vi "LINX Tasks.vi"() -> ()   [LabVIEW 2020]
doc: "This VI reads analog data from the DMA FIFO and converts it into readable signals and timestamps."
uses:
  Type Definitions/Payload Class.ctl
  Type Definitions/Enum - Data.ctl
  <vilib>/platform/TimedLoop/XDataNode/XDataNode.xnode
  <vilib>/Platform/TimedLoop/XDataNode/timing_clust.ctl
  <vilib>/Platform/TimedLoop/XDataNode/XDNodeRunTimeDep.lvlib
  <vilib>/Platform/TimedLoop/XDataNode/wakeup.ctl
  <vilib>/Platform/TimedLoop/XDataNode/nitl_modes.ctl
  <vilib>/MediaMongrels/LINX Raspberry Pi Addons/ADS1256 ADC/Channel Selection.ctl
  <vilib>/MediaMongrels/LINX Raspberry Pi Addons/LINX-DAC8552/Channel Select.ctl
  <vilib>/MediaMongrels/LINX Raspberry Pi Addons/LINX-DAC8552/Power Down Mode.ctl
  Type Definitions/Analog Output Command.ctl
  Type Definitions/Digital Output Command.ctl
  Type Definitions/Digital Output Data.ctl
  Type Definitions/Analog Output Data.ctl
  <vilib>/MakerHub/LINX/Public/Peripherals/Digital/Digital Write 1 Chan.vi
  <vilib>/MakerHub/LINX/Public/Peripherals/Digital/Digital Read N Chans.vi
panel:
  out "output cluster":T1 {"Port 0" format="%08b"}
  out "Error Out 3":errorcluster
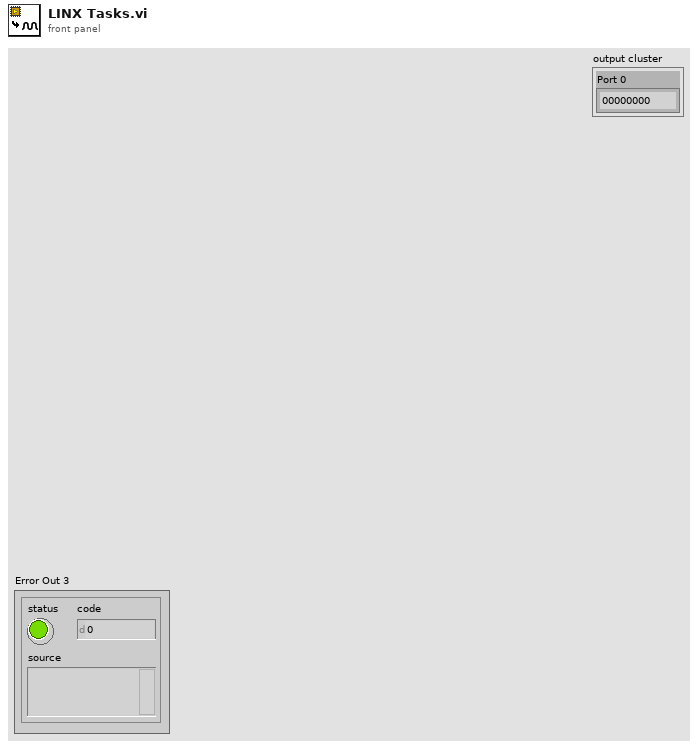
[diagram p1: front panel]
types:
  T1 = typedef "Digital Output Data.ctl" = cluster{"Port 0":u8}
  T2 = typedef "LINX-DAC8552.lvclass/Power Down Mode.ctl" = enum8{"On - Normal Operation", "Off - 1kOhm", "Off - 100kOhm", "Off - High Impedence"}
  T3 = typedef "LINX-DAC8552.lvclass/Channel Select.ctl" = enum8{"DAC A", "DAC B", "Both"}
  T4 = typedef "LINX Resources.ctl" = cluster{"LINX Resource":T5, "LINX SPI Data":refnum<class "LINX SPI.lvclass">, "ADS1256 Data":refnum<class "LINX-ADS1256.lvclass">, "DAC8552 Data":refnum<class "LINX-DAC8552.lvclass">}
  T5 = typedef "LMH-LINX.lvlib/LINX Ref.ctl" = cluster{"IO":T6, "Interface":T7, "LINX Device Config":T8}
  T6 = typedef "LMH-LINX.lvlib/Platform.ctl" = enum16{"Remote", "Local"}
  T7 = typedef "LMH-LINX.lvlib/Interface.ctl" = enum16{"Serial", "TCP"}
  T8 = typedef "LMH-LINX.lvlib/Device.lvlib/LINX Device Config.ctl" = cluster{"Interface":T7, "COM Port":refnum<visa-resource-name>, "TCP Configuration":T9, "Device Family":u8, "Device ID":u8, "Device Name":string, "TCP Ref":refnum<k5>, "Channels":T10}
  T9 = typedef "LMH-LINX.lvlib/Device.lvlib/TCP Config.ctl" = cluster{"IP Address":string, "Port":u16}
  T10 = typedef "LMH-LINX.lvlib/Channels.ctl" = cluster{"DI":u8[], "DO":u8[], "AI":u8[], "AO":u8[], "PWM":u8[], "QE":u8[], "UART":u8[], "I2C 2":u8[], "SPI":u8[], "CAN":u8[], "Servo":u8[], "AI Ref (V)":dbl, "AI Resolution (Bits)":u8, "AO Ref (V)":dbl, "AO Resolution (Bits)":u8}
  T11 = typedef "XDNodeRunTimeDep.lvlib/timing_clust.ctl" = cluster{"Expected End [f-1]":u64, "Actual End [f-1]":u64, "Finished Late? [f-1]":bool, "Expected End [i-1]":u64, "Actual End [i-1]":u64, "Finished Late? [i-1]":bool, "Expected Start [i]":u64, "Actual Start [i]":u64, "Expected Start [f]":u64, "Actual Start [f]":u64, "Source Name":string, "Structure Name":string, "Period":i64, "Deadline":i64, "Offset":i64, "Start":i64, "Priority":i32, "Timeout":i32, "Mode":T12, "Wakeup Reason":T13, "Error":errorcluster, "Source Type":string, "Secondary Source Type":string, "Global End Time":u64, "Global Start Time":u64, "Frame Duration":u64, "Iteration Duration":u64, "Assigned CPU":i32, "I/O Scan Engine Mode":u32}
  T12 = typedef "XDNodeRunTimeDep.lvlib/nitl_modes.ctl" = enum32{"No Change", "Process missed periods, maintain original phase", "Discard missed periods, maintain original phase", "Process missed periods, ignore original phase", "Discard missed periods, ignore original phase"}
  T13 = typedef "XDNodeRunTimeDep.lvlib/wakeup.ctl" = enum32{"Normal", "Aborted", "Asynchronous wakeup", "Timing source error", "Timed loop error", "Timeout"}
  T14 = typedef "Enum - Data.ctl" = enum16{"Analog Input Data", "Notification Data", "Analog Output Data", "Digital Output Data", "Command Ack", "Digital Input Data"}
  T15 = typedef "Payload Class.ctl" = enum16{"System State", "Parameters", "Metadata", "Software Monitor", "Data", "Commands"}
  T16 = typedef "Digital Output Command.ctl" = cluster{"DO Channel":u8, "State":bool}
  T17 = typedef "LINX-ADS1256.lvclass/Channel Selection.ctl" = enum16{"Differential 0-1", "Differential 2-3", "Differential 4-5", "Differential 6-7", "Single Ended 0", "Single Ended 1", "Single Ended 2", "Single Ended 3", "Single Ended 4", "Single Ended 5", "Single Ended 6", "Single Ended 7"}
  T18 = typedef "Analog Output Data.ctl" = cluster{"Bank 0":dbl[]}
  T19 = typedef "Analog Output Command.ctl" = cluster{"AO Channel":u8, "State":dbl}
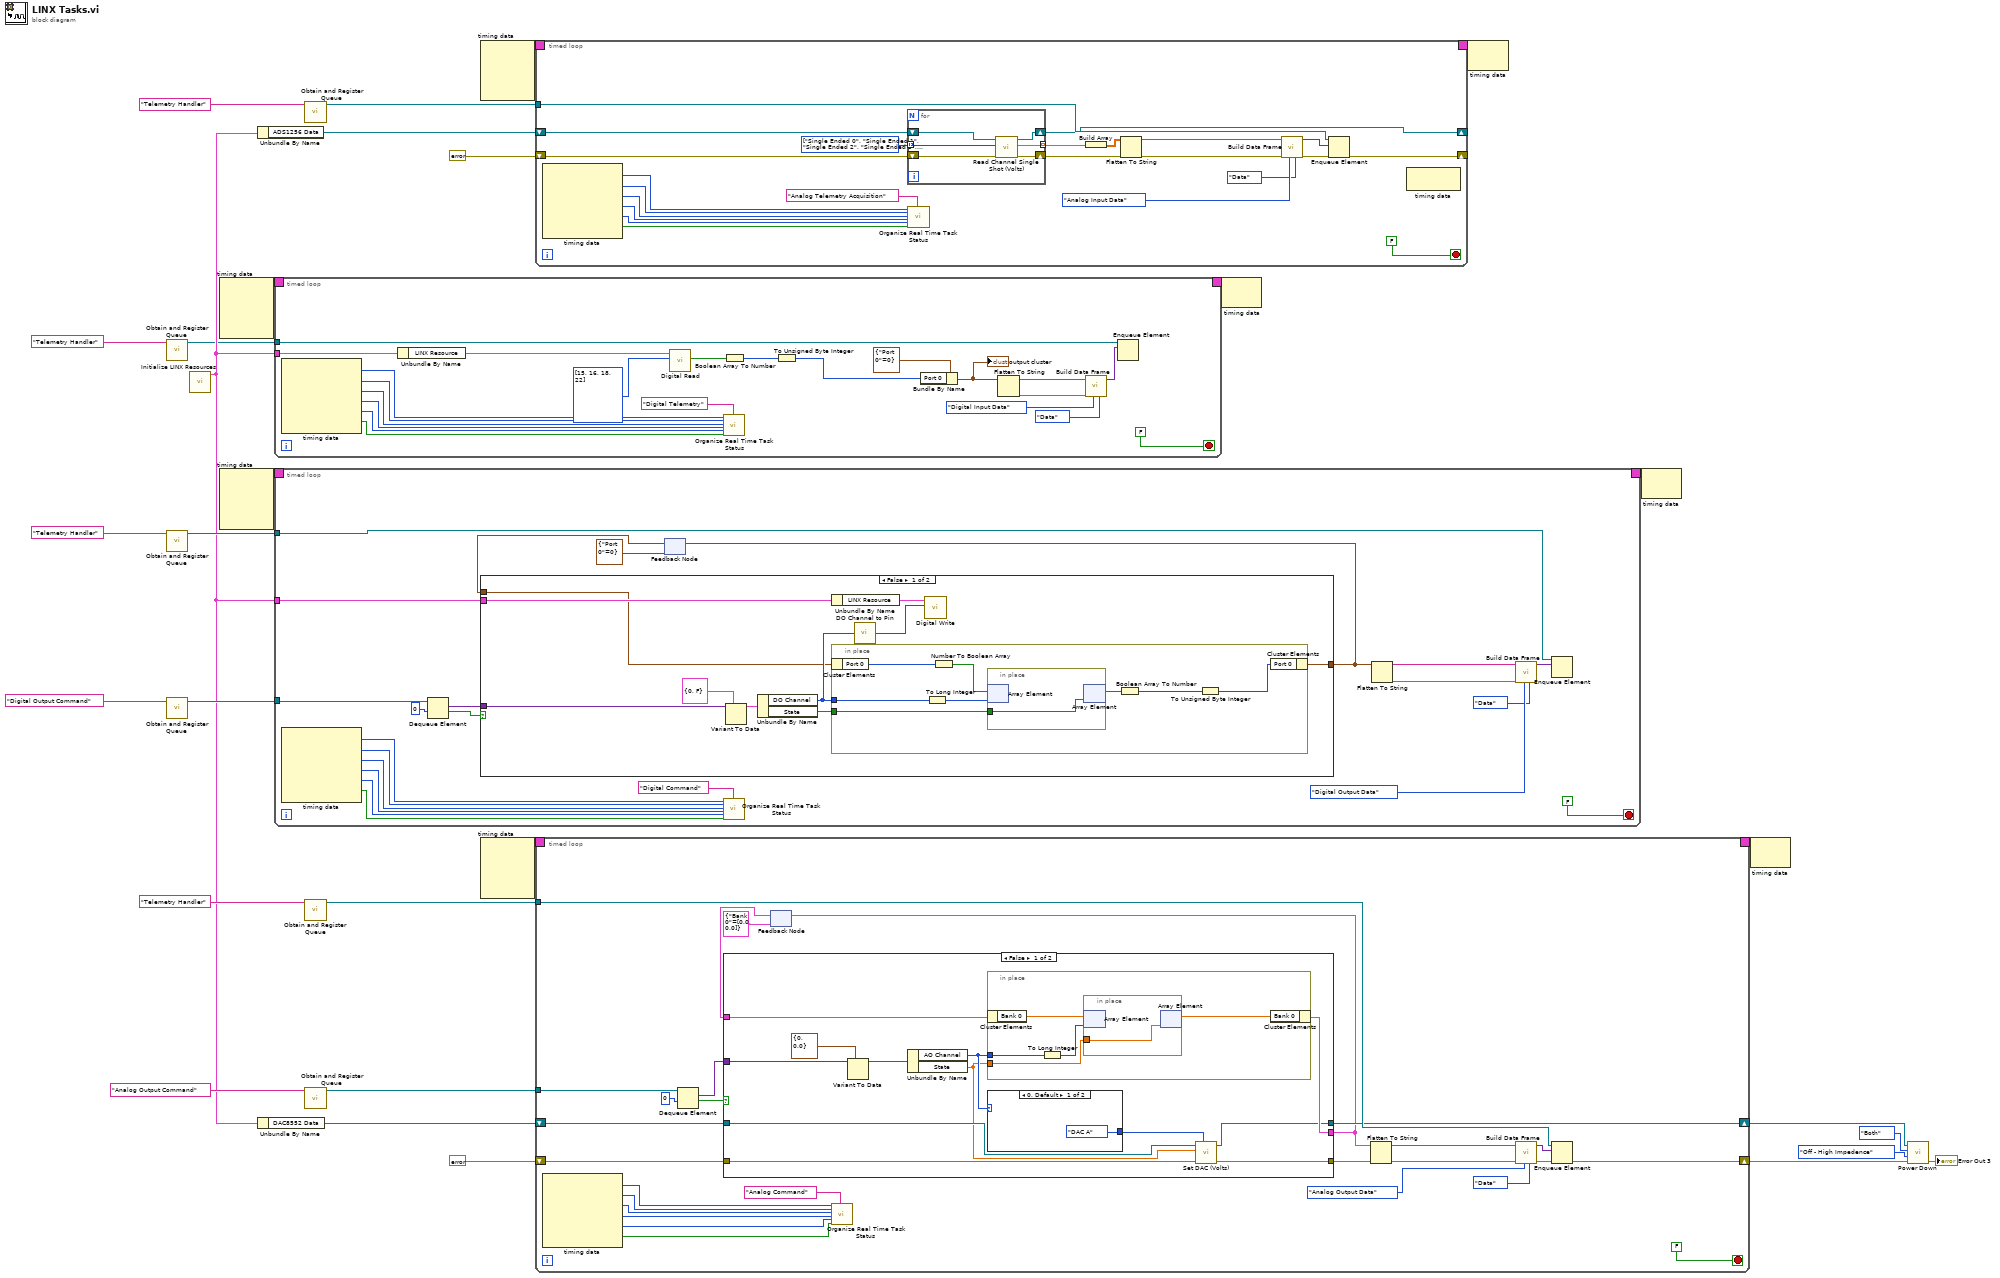
[diagram p0: block diagram]
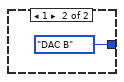
[diagram p2: hidden frame]
diagram:
  n1 = call "Obtain and Register Queue.vi"("name (unnamed)"="Telemetry Handler") -> ("Queue Out"=w1:refnum<queue>)  [unwired: 7 in, 3 out]
  n2 = call "Obtain and Register Queue.vi"("name (unnamed)"="Telemetry Handler") -> ("Queue Out"=w18:refnum<queue>)  [unwired: 7 in, 3 out]
  n3 = call "Obtain and Register Queue.vi"("name (unnamed)"="Digital Output Command") -> ("Queue Out"=w16:refnum<queue>)  [unwired: 7 in, 3 out]
  n4 = call "Initialize LINX Resources.vi"() -> ("LINX Resources"=w3:T4)  [unwired: 11 in]
  n5 = node-c288() -> (w5:T11)  [unwired: 4 in]
  n6 = node-c288() -> (w20:T11)  [unwired: 4 in]
  n7 = Unbundle By Name(w3) -> ("DAC8552 Data"=w24:refnum<class "LINX-DAC8552.lvclass">)
  n8 = Unbundle By Name(w3) -> ("ADS1256 Data"=w23:refnum<class "LINX-ADS1256.lvclass">)
  n9 = timed-loop {
    timing: w5 -> [_]
    timing-out: [_] -> w4
    tunnel: w1 -> [w38]
    tunnel: w3 -> [w44]
    stop <- FALSE stop-if-true
    n10 = node-c288() -> (w50:i32, w49:i32, w48:i64, w47:i64, w46:i64, w45:bool)  [unwired: 1 in]
    n11 = Unbundle By Name(w44) -> ("LINX Resource"=w37:T5)
    n12 = call-poly <vilib>:"Digital Read.vi"("DI Channels"=u8[] [15, 16, 18, 22] ("Array 3"), "LINX Resource"=w37) -> ("Values"=w35:bool[])  [unwired: 7 in, 2 out]
    n13 = call "Organize Real Time Task Status.vi"("Priority"=w50, "Processor"=w49, "Offset"=w48, "Iteration Duration"=w47, "Period"=w46, "Finished Late? [i-1]"=w45, "Task Name"="Digital Telemetry") -> ()  [unwired: 12 in, 1 out]
    n14 = Boolean Array To Number(Boolean array=w35) -> (number=w36:u32)
    n15 = To Unsigned Byte Integer(number=w36) -> (unsigned 8bit integer=w34:u8)
    n16 = Bundle By Name(cluster=T1 {"Port 0"=0}, "Port 0"=w34) -> (w32:T1)
    "output cluster" <- w32
    n17 = Flatten To String(anything=w32) -> (data string=w41:string, error out=w43:errorcluster)  [unwired: 3 in, 1 out]
    n18 = call "Build Data Frame.vi"("Payload Class (Data)"=Payload_Class."Data", "Payload ID (0)"=Enum_-_Data."Digital Input Data" ("Data"), "error in (no error)"=w43, "Payload (Empty String)"=w41) -> ("Frame"=w39:variant)  [unwired: 6 in, 1 out]
    n19 = Enqueue Element(queue=w38, element=w39) -> ()  [unwired: 2 in, 3 out]
  }
  n20 = timed-loop {
    timing: w20 -> [_]
    timing-out: [_] -> w19
    tunnel: w18 -> [w61]
    tunnel: w16 -> [w73]
    tunnel: w3 -> [w71]
    stop <- FALSE stop-if-true
    n21 = node-c288() -> (w80:i32, w79:i32, w78:i64, w77:i64, w76:i64, w75:bool)  [unwired: 1 in]
    n22 = Dequeue Element(queue=w73, timeout in ms (-1)=0) -> (element=w74:variant, timed out?=w70:bool)  [unwired: 1 in, 2 out]
    n23 = feedback #1(T1 {"Port 0"=0}) -> (w68:T1)
    n24 = case shown="False" w70 {
      tunnel: w74 -> [w91 _]
      tunnel: w71 -> [w89 _]
      tunnel: [w83 w102] -> w63
      tunnel: w68 -> [w84 w102]
      frame False {
        n25 = Variant To Data(type=T16 {"DO Channel"=0, "State"=FALSE}, Variant=w91) -> (data=w88:T16)  [unwired: 1 in, 1 out]
        n26 = Unbundle By Name(w88) -> ("DO Channel"=w86:u8, "State"=w85:bool)
        n27 = Unbundle By Name(w89) -> ("LINX Resource"=w90:T5)
        n28 = in-place {
          in-place-border: w86 -> [w99]
          in-place-border: w85 -> [w97]
          n29 = in-place-cluster #2(w84) -> ("Port 0"=w94:u8)
          n30 = To Long Integer(number=w99) -> (32bit integer=w98:i32)
          n31 = Number To Boolean Array(number=w94) -> (Boolean array=w100:bool[])
          n32 = in-place {
            in-place-border: w97 -> [w101]
            n33 = in-place-array #3(w100, w98) -> ()  [unwired: 1 out]
            n34 = in-place-array #3(w101) -> (w96:bool[])  [unwired: 1 out]
          }
          n35 = Boolean Array To Number(Boolean array=w96) -> (number=w95:u32)
          n36 = To Unsigned Byte Integer(number=w95) -> (unsigned 8bit integer=w93:u8)
          n37 = in-place-cluster #2("Port 0"=w93) -> (w83:T1)
        }
        n38 = call "DO Channel to Pin.vi"("DO Channel"=w86) -> ("Pin"=w87:u8)  [unwired: 4 in]
        n39 = call-poly <vilib>:"Digital Write.vi"("DO Channel"=w87, "LINX Resource"=w90) -> ()  [unwired: 8 in, 2 out]
      }
      frame True {
      }
    }
    n40 = feedback-in #1(w63) -> ()
    n41 = call "Organize Real Time Task Status.vi"("Priority"=w80, "Processor"=w79, "Offset"=w78, "Iteration Duration"=w77, "Period"=w76, "Finished Late? [i-1]"=w75, "Task Name"="Digital Command") -> ()  [unwired: 12 in, 1 out]
    n42 = Flatten To String(anything=w63) -> (data string=w65:string, error out=w67:errorcluster)  [unwired: 3 in, 1 out]
    n43 = call "Build Data Frame.vi"("Payload Class (Data)"=Payload_Class."Data", "Payload ID (0)"=Enum_-_Data."Digital Output Data" ("Data"), "error in (no error)"=w67, "Payload (Empty String)"=w65) -> ("Frame"=w62:variant)  [unwired: 6 in, 1 out]
    n44 = Enqueue Element(queue=w61, element=w62) -> ()  [unwired: 2 in, 3 out]
  }
  n45 = call "Obtain and Register Queue.vi"("name (unnamed)"="Telemetry Handler") -> ("Queue Out"=w29:refnum<queue>)  [unwired: 7 in, 3 out]
  n46 = call "Obtain and Register Queue.vi"("name (unnamed)"="Telemetry Handler") -> ("Queue Out"=w26:refnum<queue>)  [unwired: 7 in, 3 out]
  n47 = call "Obtain and Register Queue.vi"("name (unnamed)"="Analog Output Command") -> ("Queue Out"=w14:refnum<queue>)  [unwired: 7 in, 3 out]
  n48 = node-c288() -> (w28:T11)  [unwired: 4 in]
  n49 = node-c288() -> (w13:T11)  [unwired: 4 in]
  n50 = timed-loop {
    timing: w28 -> [_]
    timing-out: [_] -> w27
    tunnel: w29 -> [w123]
    shift-right: [w117] -> _
    shift-left: w23 -> [w116]
    shift-right: [w112] -> _
    shift-left: errorcluster {"status"=FALSE, "code"=0, "source"=""} ("error out") -> [w121]
    stop <- FALSE stop-if-true
    w118 = T17[] [enum."Single Ended 0", enum."Single Ended 1", enum."Single Ended 2", enum."Single Ended 3", enum."Single Ended 4", enum."Single Ended 5", enum."Single Ended 6", enum."Single Ended 7"] items=["Differential 0-1", "Differential 2-3", "Differential 4-5", "Differential 6-7", "Single Ended 0", "Single Ended 1", "Single Ended 2", "Single Ended 3", "Single Ended 4", "Single Ended 5", "Single Ended 6", "Single Ended 7"] ("Channels")
    n51 = node-c288() -> (w132:i32, w131:i32, w130:i64, w129:i64, w128:i64, w127:bool)  [unwired: 1 in]
    n52 = for "N Channels" {
      tunnel: w118 -> [w137] mode=indexing
      tunnel: [w134] -> w120 mode=indexing
      shift-right: [w136] -> w117
      shift-left: w116 -> [w139]
      shift-right: [w135] -> w115
      shift-left: w121 -> [w138]
      n53 = call <vilib>:"Read Channel Single Shot (Volts).vi"("error in (no error)"=w138, "ADC Channel Selection"=w137, "LINX-ADS1256 in"=w139) -> ("error out"=w135:errorcluster, "ADC Volts"=w134:dbl, "LINX-ADS1256 out"=w136:refnum<class "LINX-ADS1256.lvclass">)  [unwired: 6 in]
    }
    n54 = call "Organize Real Time Task Status.vi"("Priority"=w132, "Processor"=w131, "Offset"=w130, "Iteration Duration"=w129, "Period"=w128, "Finished Late? [i-1]"=w127, "Task Name"="Analog Telemetry Acquisition") -> ()  [unwired: 12 in, 1 out]
    n55 = Build Array(w120) -> (w122:dbl[][])
    n56 = Flatten To String(anything=w122, error in (no error)=w115) -> (data string=w126:string, error out=w114:errorcluster)  [unwired: 2 in, 1 out]
    n57 = call "Build Data Frame.vi"("Payload Class (Data)"=Payload_Class."Data", "Payload ID (0)"=Enum_-_Data."Analog Input Data" ("Data"), "error in (no error)"=w114, "Payload (Empty String)"=w126) -> ("error out"=w113:errorcluster, "Frame"=w124:variant)  [unwired: 6 in]
    n58 = Enqueue Element(queue=w123, element=w124, error in (no error)=w113) -> (error out=w112:errorcluster)  [unwired: 1 in, 2 out]
    n59 = node-c288() -> ()  [unwired: 1 in, 1 out]
  }
  n60 = timed-loop {
    timing: w13 -> [_]
    timing-out: [_] -> w12
    tunnel: w26 -> [w158]
    shift-right: [w157] -> w11
    shift-left: errorcluster {"status"=FALSE, "code"=0, "source"=""} ("error out") -> [w166]
    shift-right: [w153] -> w10
    shift-left: w24 -> [w165]
    tunnel: w14 -> [w156]
    stop <- FALSE stop-if-true
    n61 = node-c288() -> (w172:i32, w171:i32, w170:i64, w169:i64, w168:i64, w167:bool)  [unwired: 1 in]
    n62 = Dequeue Element(queue=w156, timeout in ms (-1)=0) -> (element=w154:variant, timed out?=w148:bool)  [unwired: 1 in, 2 out]
    n63 = feedback #4(T18 {"Bank 0"=[0.0, 0.0]}) -> (w150:T18)
    n64 = case shown="False" w148 {
      tunnel: w166 -> [w186 w195]
      tunnel: w165 -> [w185 w196]
      tunnel: w154 -> [w182 _]
      tunnel: [w176 w196] -> w153
      tunnel: [w175 w195] -> w152
      tunnel: w150 -> [w177 w197]
      tunnel: [w178 w197] -> w149
      frame False {
        n65 = Variant To Data(type=T19 {"AO Channel"=0, "State"=0.0} ("Analog Output Command"), Variant=w182) -> (data=w183:T19)  [unwired: 1 in, 1 out]
        n66 = Unbundle By Name(w183) -> ("AO Channel"=w180:u8, "State"=w179:dbl)
        n67 = in-place {
          in-place-border: w180 -> [w190]
          in-place-border: w179 -> [w188]
          n68 = in-place-cluster #5(w177) -> ("Bank 0"=w191:dbl[])
          n69 = To Long Integer(number=w190) -> (32bit integer=w189:i32)
          n70 = in-place {
            in-place-border: w188 -> [w192]
            n71 = in-place-array #6(w191, w189) -> ()  [unwired: 1 out]
            n72 = in-place-array #6(w192) -> (w187:dbl[])  [unwired: 1 out]
          }
          n73 = in-place-cluster #5("Bank 0"=w187) -> (w178:T18)
        }
        n74 = case shown="0, Default" w180 {
          tunnel: [Channel_Select."DAC A" ("Channel Select") Channel_Select."DAC B" ("Channel Select")] -> w181
          frame 0, Default {
          }
          frame 1 {
          }
        }
        n75 = call <vilib>:"Set DAC (Volts).vi"("Channel Select"=w181, "error in (no error)"=w186, "DAC Output (V)"=w179, "DAC8552 in"=w185) -> ("error out"=w175:errorcluster, "DAC8552 out"=w176:refnum<class "LINX-DAC8552.lvclass">)  [unwired: 6 in]
      }
      frame True {
      }
    }
    n76 = feedback-in #4(w149) -> ()
    n77 = call "Organize Real Time Task Status.vi"("Priority"=w172, "Processor"=w171, "Offset"=w170, "Iteration Duration"=w169, "Period"=w168, "Finished Late? [i-1]"=w167, "Task Name"="Analog Command") -> ()  [unwired: 12 in, 1 out]
    n78 = Flatten To String(anything=w149, error in (no error)=w152) -> (data string=w163:string, error out=w160:errorcluster)  [unwired: 2 in, 1 out]
    n79 = call "Build Data Frame.vi"("Payload Class (Data)"=Payload_Class."Data", "Payload ID (0)"=Enum_-_Data."Analog Output Data" ("Data"), "error in (no error)"=w160, "Payload (Empty String)"=w163) -> ("error out"=w159:errorcluster, "Frame"=w161:variant)  [unwired: 6 in]
    n80 = Enqueue Element(queue=w158, element=w161, error in (no error)=w159) -> (error out=w157:errorcluster)  [unwired: 1 in, 2 out]
  }
  n81 = node-c288(w4) -> ()  [unwired: 1 out]
  n82 = node-c288(w27) -> ()  [unwired: 1 out]
  n83 = node-c288(w19) -> ()  [unwired: 1 out]
  n84 = node-c288(w12) -> ()  [unwired: 1 out]
  n85 = call <vilib>:"Power Down.vi"("error in (no error)"=w11, "Power Down Mode"=Power_Down_Mode."Off - High Impedence", "Channel Select"=Channel_Select."Both", "DAC8552 in"=w10) -> ("error out"=→"Error Out 3":errorcluster)  [unwired: 6 in, 1 out]
